vi "Launch Configured Tasks.vi"(8 "error in (no error)":errorcluster, 11 "VolatusCore in":refnum<class "VolatusCore.lvclass">) -> (0 "error out":errorcluster, 3 "VolatusCore out":refnum<class "VolatusCore.lvclass">)   [LabVIEW 2020, in "Volatus.lvlib" / "VolatusCore.lvclass"]
uses:
  VolatusCore.lvclass
  VolatusCore.lvclass/VolatusCore.ctl
  VolatusConfig/Node/Node.lvclass
  VolatusConfig/Task/Task.lvclass
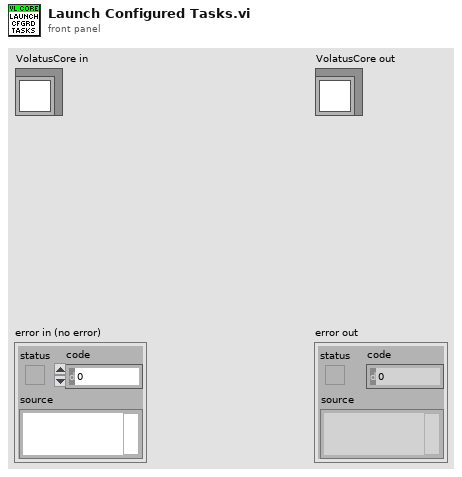
[diagram p1: front panel]
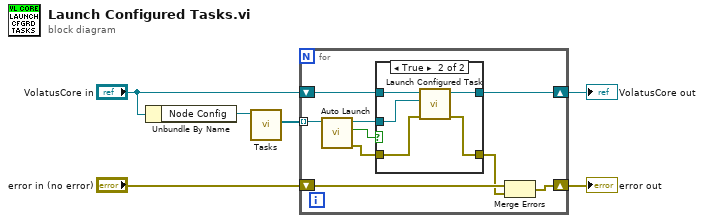
[diagram p0: block diagram]
diagram:
  n1 = Unbundle By Name("VolatusCore in") -> ("Node Config"=w6:refnum<class "Node.lvclass">)
  n2 = call "Tasks.vi"("Node in"=w6) -> ("Tasks"=w4:refnum<class "Task.lvclass">[])  [unwired: 8 in, 2 out]
  n3 = for {
    shift-right: [w9] -> w2
    shift-left: "VolatusCore in" -> [w8]
    tunnel: w4 -> [w15] mode=indexing
    shift-right: [w10] -> w1
    shift-left: "error in (no error)" -> [w12]
    n4 = call "Auto Launch.vi"("Task in"=w15) -> ("error out"=w13:errorcluster, "Auto Launch"=w14:bool, "Task out"=w7:refnum<class "Task.lvclass">)  [unwired: 8 in]
    n5 = case shown="True" w14 {
      tunnel: w13 -> [w17 w19]
      tunnel: [w17 w18] -> w11
      tunnel: [w16 w20] -> w9
      tunnel: w8 -> [w16 w22]
      tunnel: w7 -> [_ w21]
      frame False {
      }
      frame True {
        n6 = call "Launch Configured Task.vi"("error in (no error)"=w19, "Task"=w21, "VolatusCore in"=w22) -> ("error out"=w18:errorcluster, "VolatusCore out"=w20:refnum<class "VolatusCore.lvclass">)  [unwired: 7 in]
      }
    }
    n7 = Merge Errors(w12, w11) -> (w10:errorcluster)
  }
  "error out" <- w1
  "VolatusCore out" <- w2
